vi "2011 Vision Example_3061.vi"() -> ()   [LabVIEW 2011]
doc: "This example shows how to use color threshold, filtering, and particle analysis to locate reflective tape."
uses:
  <vilib>/vision/NI_Vision_Development_Module.lvlib
panel:
  in  "Add to Checlk":bool
  out "Waveform Chart":dbl(graph)
  in  "method":enum16{"2 points", "4 points"}(ring)
  in  "Tab Control":enum32{"Page 1", "Page 2"}(tab)
  out "Distance":dbl[](array[numeric])=[12.237087490204587] format="%#.2f"
  in  "Hoop Height":dbl=5.8
  in  "Camera Height":dbl=4.0
  in  "Y":dbl=10.0
  in  "X":dbl
  out "True Distance":dbl=10.16070863670443 format="%_4g"
  out "Distance Error (%)":dbl=20.435374418664757 format="%.2f"
  out "Distance Error (ft)":dbl=2.0763788535001577 format="%.2f"
  out "4Side Length":dbl[](array[numeric])=[49.431228982320626, 66.27846474701015, 49.519367071613864, 66.23966390572282]
  out "dH":dbl=-0.08813808929323841
  out "dW":dbl=0.03880084128732619
  out "Original Image 2":T1(plugin-control)
  out "Particle (Pixels)":dbl[][](array[numeric])=[[203.0, 71.0, 60.0, 53.0]] format="%.2f"
  in  "Stop":bool
  out "4 corners Image":T1(plugin-control)
  in  "path":path=path "C:/Documents and Settings/u00ixr7/Desktop/3061 hoop pics"
  out "Masked Image":T1(plugin-control)
  out "Original Image":T1(plugin-control)
  in  "Files":i32(listbox)=6
  in  "Luma Range":cluster{"Lower value":i32, "Upper value":i32}={"Lower value"=20, "Upper value"=1000}
  in  "Sat Range":cluster{"Lower value":i32, "Upper value":i32}={"Lower value"=80, "Upper value"=1000}
  in  "Hue Range":cluster{"Lower value":i32, "Upper value":i32}={"Lower value"=100, "Upper value"=1000}
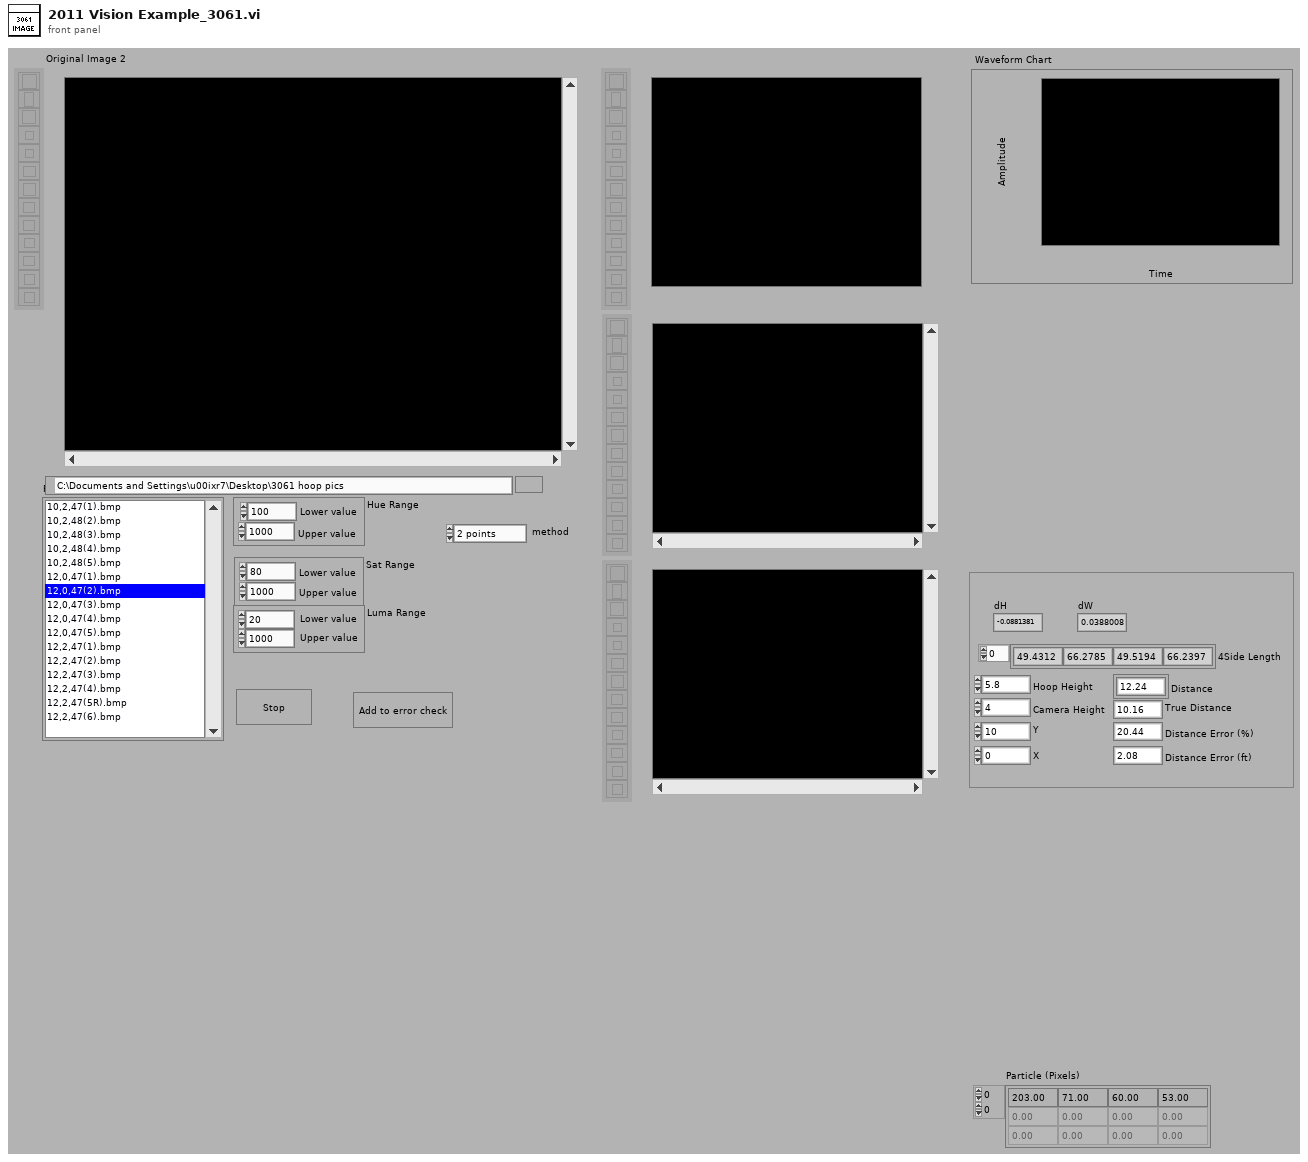
[diagram p1: front panel]
types:
  T1 = typedef "IMAQ Image.ctl" = refnum<image>
  T2 = typedef "Image Type" = u32
  T3 = typedef "Particle Parameters" = i32
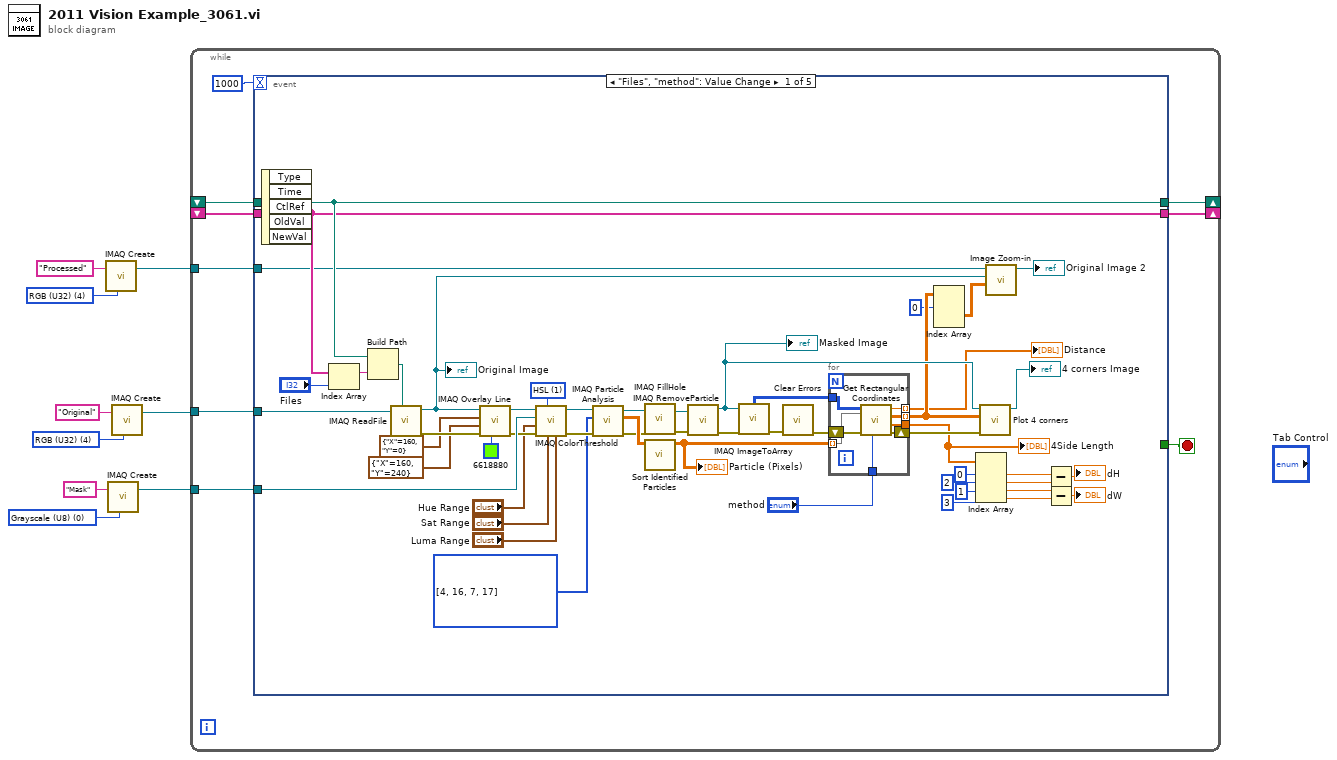
[diagram p0: block diagram]
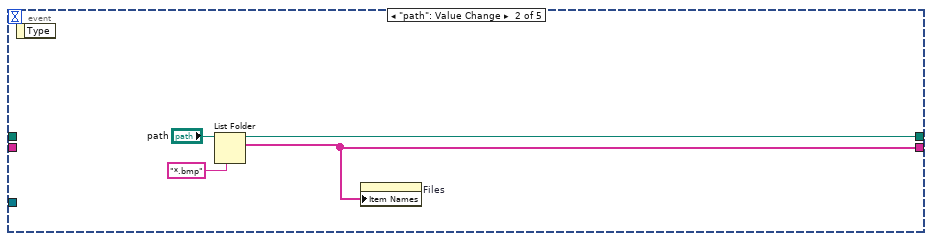
[diagram p2: hidden frame]
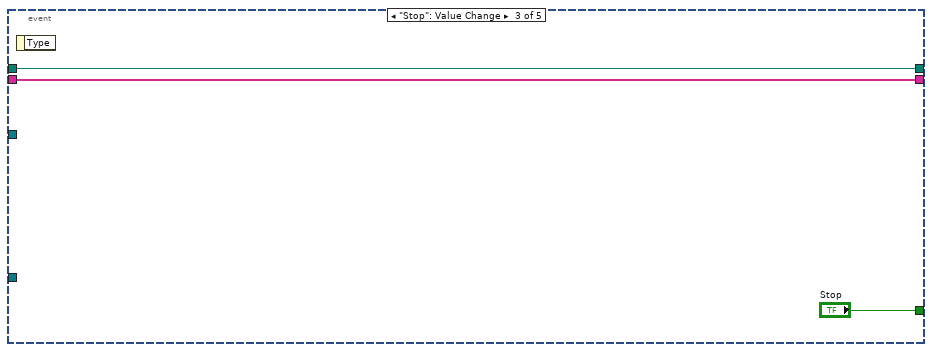
[diagram p3: hidden frame]
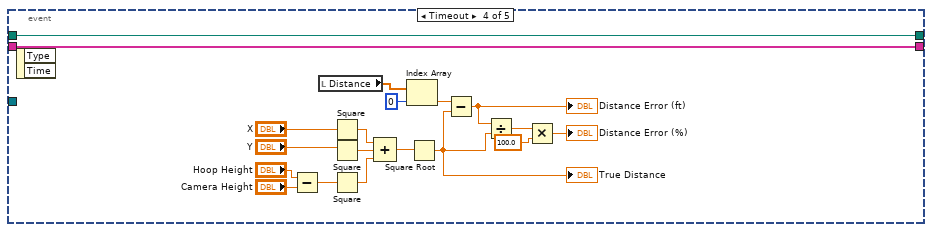
[diagram p4: hidden frame]
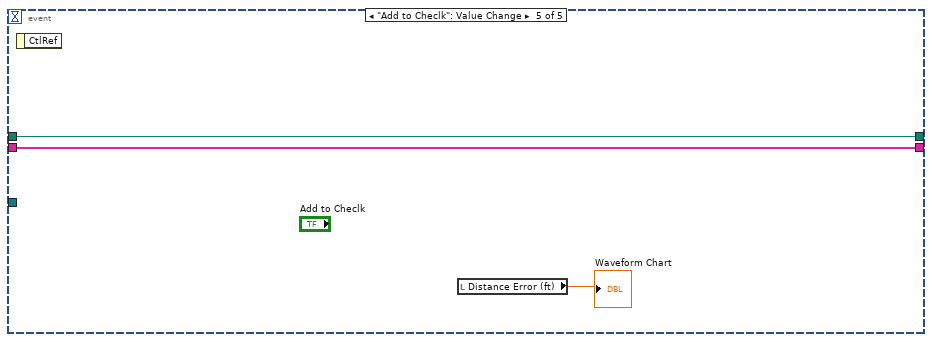
[diagram p5: hidden frame]
diagram:
  w3 = T2 4 items=["Grayscale (U8)", "Grayscale (I16)", "Grayscale (SGL)", "Complex (CSG)", "RGB (U32)", "HSL (U32)", "RGB (U64)", "Grayscale (U16)"] ("Image Type")
  w6 = T2 0 items=["Grayscale (U8)", "Grayscale (I16)", "Grayscale (SGL)", "Complex (CSG)", "RGB (U32)", "HSL (U32)", "RGB (U64)", "Grayscale (U16)"] ("Image Type")
  w8 = T2 4 items=["Grayscale (U8)", "Grayscale (I16)", "Grayscale (SGL)", "Complex (CSG)", "RGB (U32)", "HSL (U32)", "RGB (U64)", "Grayscale (U16)"] ("Image Type")
  n1 = call "IMAQ Create"("Image Name"="Processed", "Image Type"=w3) -> ("New Image"=w1:T1)  [unwired: 2 in, 2 out]
  n2 = call "IMAQ Create"("Image Name"="Mask", "Image Type"=w6) -> ("New Image"=w4:T1)  [unwired: 2 in, 2 out]
  n3 = call "IMAQ Create"("Image Name"="Original", "Image Type"=w8) -> ("New Image"=w7:T1)  [unwired: 2 in, 2 out]
  n4 = while {
    tunnel: w7 -> [w18]
    tunnel: w4 -> [w16]
    shift-right: [w13] -> _
    shift-left: _ -> [w17]
    shift-right: [w12] -> _
    shift-left: _ -> [w15]
    tunnel: w1 -> [w10]
    stop <- w14 stop-if-true
    n5 = event shown="[0] \"Files\", \" method\": Value Change" {
      selector: _ -> [_ _ _ _ _]
      dyn-events: _ -> [_ _ _ _ _]
      timeout: 1000 -> [_ _ _ _ _]
      tunnel: w18 -> [w69 _ _ _ _]
      tunnel: w17 -> [w32 _ w82 w85 w106]
      tunnel: w16 -> [w68 _ _ _ _]
      tunnel: w15 -> [w31 _ w83 w86 w105]
      tunnel: [_ _ "Stop" _ _] -> w14
      tunnel: [w32 w79 w82 w85 w106] -> w13
      tunnel: [w31 w78 w83 w86 w105] -> w12
      tunnel: w10 -> [w30 _ _ _ _]
      event "Files", "method": Value Change {
        w57 = T3[] [4, 16, 7, 17] items=["Center of Mass X", "Center of Mass Y", "First Pixel X", "First Pixel Y", "Bounding Rect Left", "Bounding Rect Top", "Bounding Rect Right", "Bounding Rect Bottom", "Max Feret Diameter Start X", "Max Feret Diameter Start Y", "Max Feret Diameter End X", "Max Feret Diameter End Y", "Max Horiz. Segment Length Left", "Max Horiz. Segment Length Right", "Max Horiz. Segment Length Row", "-", "Bounding Rect Width", "Bounding Rect Height", "Bounding Rect Diagonal", "Perimeter", "Convex Hull Perimeter", "Holes' Perimeter", "Max Feret Diameter", "Equivalent Ellipse Major Axis", "Equivalent Ellipse Minor Axis", "Equivalent Ellipse Minor Axis (Feret)", "Equivalent Rect Long Side", "Equivalent Rect Short Side", "Equivalent Rect Diagonal", "Equivalent Rect Short Side (Feret)", "Average Horiz. Segment Length", "Average Vert. Segment Length", "Hydraulic Radius", "Waddel Disk Diameter", "-", "Area", "Holes' Area", "Particle & Holes' Area", "Convex Hull Area", "Image Area", "-", "Number of Holes", "Number of Horiz. Segments", "Number of Vert. Segments", "-", "Orientation", "Max Feret Diameter Orientation", "-", "% Area/Image Area", "% Area/(Particle & Holes' Area)", "Ratio of Equivalent Ellipse Axes", "Ratio of Equivalent Rect Sides", "-", "Elongation Factor", "Compactness Factor", "Heywood Circularity Factor", "Type Factor", "-", "Sum X", "Sum Y", "Sum XX", "Sum XY", "Sum YY", "Sum XXX", "Sum XXY", "Sum XYY", "Sum YYY", "-", "Moment of Inertia XX", "Moment of Inertia XY", "Moment of Inertia YY", "Moment of Inertia XXX", "Moment of Inertia XXY", "Moment of Inertia XYY", "Moment of Inertia YYY", "Norm. Moment of Inertia XX", "Norm. Moment of Inertia XY", "Norm. Moment of Inertia YY", "Norm. Moment of Inertia XXX", "Norm. Moment of Inertia XXY", "Norm. Moment of Inertia XYY", "Norm. Moment of Inertia YYY", "Hu Moment 1", "Hu Moment 2", "Hu Moment 3", "Hu Moment 4", "Hu Moment 5", "Hu Moment 6", "Hu Moment 7"] ("subarray")
        w62 = u16 1 items=["RGB", "HSL", "HSV", "HSI"] ("Color Mode")
        n6 = event-data() -> ()  [unwired: 1 in, 5 out]
        n7 = Index Array(array=w31, index="Files") -> (element=w46:string)
        n8 = Build Path(base path=w32, name or relative path=w46) -> (appended path=w67:path)
        n9 = call "IMAQ ReadFile"("File Path"=w67, "Image"=w69) -> ("error out"=w66:errorcluster, "Image Out"=w24:T1)  [unwired: 3 in, 5 out]
        "Original Image" <- w24
        n10 = call "IMAQ Overlay Line"("Color"=u32 6618880, "End Point"=cluster{"X":i32, "Y":i32} {"X"=160, "Y"=240}, "Start Point"=cluster{"X":i32, "Y":i32} {"X"=160, "Y"=0}, "Image"=w24) -> ("Image Out"=w26:T1)  [unwired: 6 in, 1 out]
        n11 = call "IMAQ ColorThreshold"("Blue or Luma or Val or Inten Range"="Luma Range", "Green or Sat Range"="Sat Range", "Color Mode"=w62, "error in (no error)"=w66, "Red or Hue Range"="Hue Range", "Image Dst"=w68, "Image Src"=w26) -> ("error out"=w61:errorcluster, "Image Dst Out"=w60:T1)  [unwired: 1 in, 2 out]
        n12 = call "IMAQ Particle Analysis"("error in (no error)"=w61, "Pixel Measurements"=w57, "Image"=w60) -> ("error out"=w56:errorcluster, "Particle Measurements (Pixels)"=w58:dbl[][], "Image Out (duplicate)"=w59:T1)  [unwired: 2 in, 4 out]
        n13 = call "IMAQ FillHole"("error in (no error)"=w56, "Image Src"=w59) -> ("error out"=w53:errorcluster, "Image Dst Out"=w51:T1)  [unwired: 4 in]
        n14 = call "Sort Identified Particles.vi"("Particle (Pixels)"=w58) -> ("Particle (Pixels)out"=w44:dbl[][])  [unwired: 10 in]
        "Particle (Pixels)" <- w44
        n15 = call "IMAQ RemoveParticle"("error in (no error)"=w53, "Image Src"=w51) -> ("error out"=w52:errorcluster, "Image Dst Out"=w48:T1)  [unwired: 8 in]
        "Masked Image" <- w48
        n16 = call "IMAQ ImageToArray"("error in (no error)"=w52, "Image"=w48) -> ("error out"=w55:errorcluster, "Image Pixels (U8)"=w50:u8[][])  [unwired: 2 in, 3 out]
        n17 = call <vilib>:"Clear Errors.vi"("error in (no error)"=w55) -> ("error out"=w54:errorcluster)  [unwired: 6 out]
        n18 = for {
          tunnel: w50 -> [w76]
          tunnel: [w75] -> w23 mode=indexing
          tunnel: [w73] -> w20 mode=indexing
          tunnel: w44 -> [w72] mode=indexing
          shift-right: [w74] -> w47
          shift-left: w54 -> [w77]
          tunnel: [w71] -> w43
          tunnel: "method" -> [w70]
          n19 = call "Get Rectangular Coordinates.vi"("method"=w70, "error in (no error)"=w77, "Particle Measurements (Pixels)"=w72, "Image Pixels (U8)"=w76) -> ("error out"=w74:errorcluster, "4Side Length"=w71:dbl[], "4 corner Coordinates"=w75:dbl[][], "Distance (ft)"=w73:dbl)  [unwired: 4 in]
        }
        "Distance" <- w20
        "4Side Length" <- w43
        n20 = Index Array(array=w23, index (dim 0)=0 ("index (page)")) -> (element=w21:dbl[][])  [unwired: 2 in]
        n21 = Index Array(array=w43, index #1=0 ("index"), index #2=2 ("index"), index #3=1 ("index"), index #4=3 ("index")) -> (element #1=w37:dbl, element #2=w38:dbl, element #3=w36:dbl, element #4=w35:dbl)
        n22 = call "Plot 4 corners.vi"("error in (no error)"=w47, "4 corners"=w23, "Refnum in"=w48) -> ("Refnum out"=→"4 corners Image":T1)  [unwired: 7 in, 1 out]
        n23 = call "Image Zoom-in.vi"("4 corners"=w21, "Original"=w24, "Processed"=w30) -> ("Processed out"=→"Original Image 2":T1)  [unwired: 7 in, 1 out]
        n24 = Subtract(x=w37, y=w38) -> (x-y=→"dH":dbl)
        n25 = Subtract(x=w36, y=w35) -> (x-y=→"dW":dbl)
      }
      event "path": Value Change {
        n26 = event-data() -> ()  [unwired: 1 in, 1 out]
        n27 = List Folder(path="path", pattern="*.bmp") -> (path out=w79:path, filenames=w78:string[])  [unwired: 1 in, 3 out]
        n28 = property on="Files" class="LstBox (strict)"("Item Names"=w78) -> ()  [unwired: 2 in, 2 out]
      }
      event "Stop": Value Change {
        n29 = event-data() -> ()  [unwired: 1 in, 1 out]
      }
      event Timeout {
        n30 = event-data() -> ()  [unwired: 1 in, 2 out]
        n31 = Subtract(x="Hoop Height", y="Camera Height") -> (x-y=w101:dbl)
        n32 = local read "Distance"() -> (w94:dbl[])
        n33 = Square(x="X") -> (x^2=w98:dbl)
        n34 = Square(x="Y") -> (x^2=w97:dbl)
        n35 = Square(x=w101) -> (x^2=w96:dbl)
        n36 = Compound Arithmetic op=ADD(w98, w97, w96) -> (w95:dbl)
        n37 = Index Array(array=w94, index=0) -> (element=w92:dbl)
        n38 = Square Root(x=w95) -> (sqrt(x)=w90:dbl)
        "True Distance" <- w90
        n39 = Subtract(x=w92, y=w90) -> (x-y=w91:dbl)
        "Distance Error (ft)" <- w91
        n40 = Divide(x=w91, y=w90) -> (x/y=w89:dbl)
        n41 = Multiply(x=w89, y=100.0) -> (x*y=→"Distance Error (%)":dbl)
      }
      event "Add to Checlk": Value Change {
        n42 = event-data() -> ()  [unwired: 1 in, 1 out]
        n43 = local read "Distance Error (ft)"() -> (→"Waveform Chart":dbl)
      }
    }
  }
